vi "PathPlanner_Point_Equals.vi"(9 "Other GoalEndState":T1={"Position"={"X"=0.0, "Y"=0.0}, "HolonomicRotation"={"VALUE"=0.0, "COS"=1.0, "SIN"=0.0}, "DistAlongPath"=0.0, "CurveRadius"=0.0, "MaxV"=9e+300, "Constraints"={"MaxVelocityMps;"=0.0, "MaxAccelerationMpsSq;"=0.0, "MaxAngularVelRadPsEc;"=0.0, "MaxAngularAccRadPSecSq"=0.0}, "HolonomicRotationExists"=FALSE} {"HolonomicRotation"."SIN" format="%13.4f"; "HolonomicRotation"."COS" format="%13.4f"; "HolonomicRotation"."VALUE" format="%13.4f"; "Position"."Y" format="%14.3f"; "Position"."X" format="%14.3f"}, 11 "PathPlannerPoint":T1={"Position"={"X"=0.0, "Y"=0.0}, "HolonomicRotation"={"VALUE"=0.0, "COS"=1.0, "SIN"=0.0}, "DistAlongPath"=0.0, "CurveRadius"=0.0, "MaxV"=9e+300, "Constraints"={"MaxVelocityMps;"=0.0, "MaxAccelerationMpsSq;"=0.0, "MaxAngularVelRadPsEc;"=0.0, "MaxAngularAccRadPSecSq"=0.0}, "HolonomicRotationExists"=FALSE} {"HolonomicRotation"."SIN" format="%13.4f"; "HolonomicRotation"."COS" format="%13.4f"; "HolonomicRotation"."VALUE" format="%13.4f"; "Position"."Y" format="%14.3f"; "Position"."X" format="%14.3f"}) -> (3 "Equal":bool)   [LabVIEW 2019, in "PathPlanner24.lvlib"]
doc: "/**\n * Create a new path constraints object\n *\n * @param maxVelocityMps Max linear velocity (M/S)\n * @param maxAccelerationMpsSq Max linear acceleration (M/S^2)\n * @param maxAngularVelocityRps Max angular velocity (Rad/S)\n * @param maxAngularAccelerationRpsSq Max angular acceleration (Rad/S^2)\n */"
uses:
  PathPlanner24.lvlib
  <vilib>/Rock Robotics/WPI/ThirdParty/JAS_Junk/TrajLib/Trajectory_Library.lvlib
  <vilib>/Rock Robotics/WPI/ThirdParty/JAS_Junk/TrajLib/TypeDef/ROTATION2D.ctl
  <vilib>/Rock Robotics/WPI/ThirdParty/JAS_Junk/TrajLib/TypeDef/TRANSLATION2D.ctl
  TypeDef/PathPlannerPathConstraints.ctl
  TypeDef/PathPlannerPoint.ctl
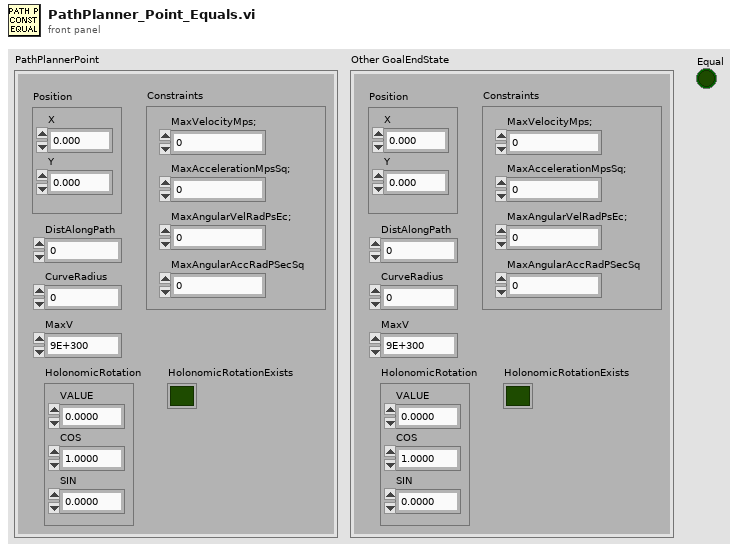
[diagram p1: front panel]
types:
  T1 = typedef "PathPlanner24.lvlib/PathPlannerPoint.ctl" = cluster{"Position":T2, "HolonomicRotation":T3, "DistAlongPath":dbl, "CurveRadius":dbl, "MaxV":dbl, "Constraints":T4, "HolonomicRotationExists":bool}
  T2 = typedef "Trajectory_Library.lvlib/TRANSLATION2D.ctl" = cluster{"X":dbl, "Y":dbl}
  T3 = typedef "Trajectory_Library.lvlib/ROTATION2D.ctl" = cluster{"VALUE":dbl, "COS":dbl, "SIN":dbl}
  T4 = typedef "PathPlanner24.lvlib/PathPlannerPathConstraints.ctl" = cluster{"MaxVelocityMps;":dbl, "MaxAccelerationMpsSq;":dbl, "MaxAngularVelRadPsEc;":dbl, "MaxAngularAccRadPSecSq":dbl}
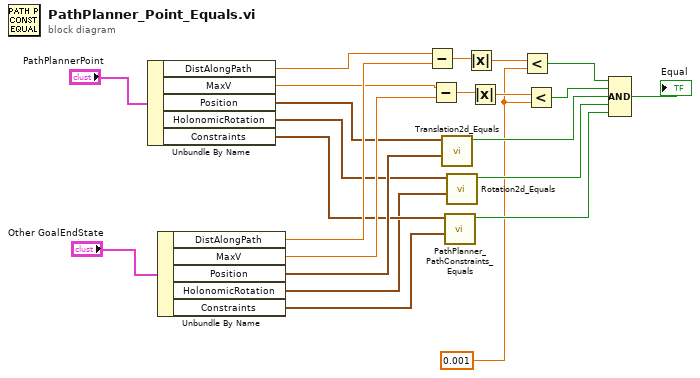
[diagram p0: block diagram]
diagram:
  w1 = 0.001 ("y")
  n1 = Unbundle By Name("PathPlannerPoint") -> ("DistAlongPath"=w21:dbl, "MaxV"=w13:dbl, "Position"=w10:T2, "HolonomicRotation"=w8:T3, "Constraints"=w7:T4)
  n2 = Unbundle By Name("Other GoalEndState") -> ("DistAlongPath"=w20:dbl, "MaxV"=w12:dbl, "Position"=w9:T2, "HolonomicRotation"=w6:T3, "Constraints"=w5:T4)
  n3 = Subtract(x=w21, y=w20) -> (x-y=w19:dbl)
  n4 = Subtract(x=w13, y=w12) -> (x-y=w15:dbl)
  n5 = call <vilib>:"Translation2d_Equals.vi"("other Translation"=w9, "In Translation"=w10) -> ("Equals"=w4:bool)  [unwired: 9 in]
  n6 = call "PathPlanner_PathConstraints_Equals.vi"("Other PathPlannerConstraints"=w5, "PathPlannerConstraints"=w7) -> ("Equal"=w2:bool)  [unwired: 9 in]
  n7 = call <vilib>:"Rotation2d_Equals.vi"("other ROTATION"=w6, "in ROTATION"=w8) -> ("Equals"=w3:bool)  [unwired: 9 in]
  n8 = Absolute Value(x=w19) -> (abs(x)=w18:dbl)
  n9 = Absolute Value(x=w15) -> (abs(x)=w14:dbl)
  n10 = Less?(x=w18, y=w1) -> (x < y?=w17:bool)
  n11 = Less?(x=w14, y=w1) -> (x < y?=w11:bool)
  n12 = Compound Arithmetic op=AND(w17, w11, w4, w3, w2) -> (→"Equal":bool)
